vi "Plot Name Creator.vi"(1 "clsData":T1) -> (0 "plotName":string)   [LabVIEW 2013]
doc: "This VI will compile deatils of the plot into a string."
uses:
  controls/clsData.ctl
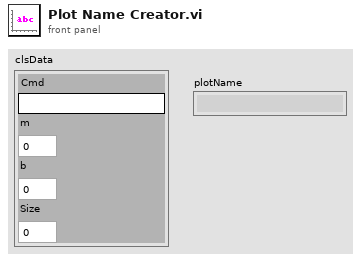
[diagram p1: front panel]
types:
  T1 = typedef "clsData.ctl" = cluster{"Cmd":string, "m":dbl, "b":dbl, "Size":u32}
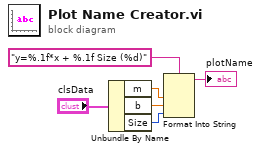
[diagram p0: block diagram]
diagram:
  n1 = Unbundle By Name("clsData") -> ("m"=w4:dbl, "b"=w3:dbl, "Size"=w2:u32)
  n2 = Format Into String(format string="y=%.1f*x + %.1f Size (%d)", w4, w3, w2) -> (resulting string=→"plotName":string)  [unwired: 2 in, 1 out]
